vi "MB Serial Master Query Read Input Registers (poly).vi"(0 "VISA resource name":refnum<visa-resource-name>, 1 "Starting Address":u16, 2 "Quantity":u16=1, 4 "Timeout":u32=5000, 5 "error in":errorcluster, 6 "Serial Parameters":T1 {"Slave Address" format="%.0x"}) -> (14 "VISA resource name out":refnum<visa-resource-name>, 15 "Input Registers":u16[](array[numeric]), 16 "Exception Code":u8 format="%.0x", 19 "error out":errorcluster)   [LabVIEW 2011]
doc: "The master uses this VI to read the slaves input registers. This corresponds to a public function code of 4 in the MODBUS protocol."
uses:
  MB Modbus Command.ctl
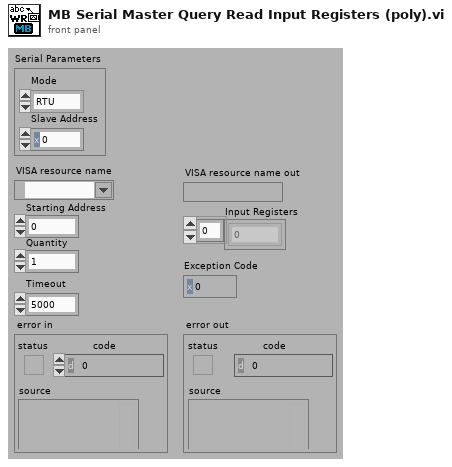
[diagram p1: front panel]
types:
  T1 = cluster{"Mode":enum16{"RTU", "ASCII"}, "Slave Address":u8}
  T2 = typedef "MB Modbus Command.ctl" = cluster{"Function Code":u8, "Starting Address":u16, "Quantity":u16, "Data":u16[], "Discrete":bool[]}
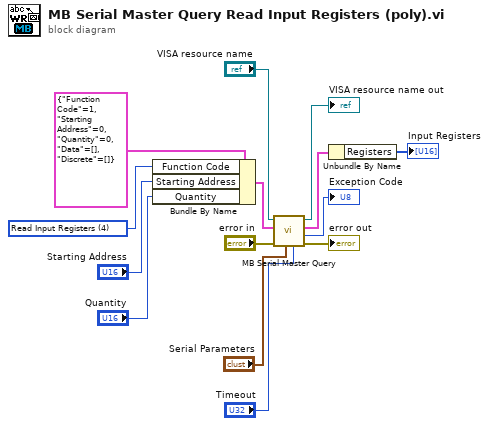
[diagram p0: block diagram]
diagram:
  w11 = u8 4 items=["Read Coils"=1, "Read Discrete Inputs"=2, "Read Holding Registers"=3, "Read Input Registers"=4, "Write Single Coil"=5, "Write Single Register"=6, "Read Exception Status"=7, "Write Multiple Coils"=15, "Write Multiple Registers"=16] ("Function Code")
  n1 = Bundle By Name(cluster=T2 {"Function Code"=1, "Starting Address"=0, "Quantity"=0, "Data"=[], "Discrete"=[]} ("Modbus Command"), "Function Code"=w11, "Starting Address"="Starting Address", "Quantity"="Quantity") -> (w12:T2)
  n2 = call "MB Serial Master Query.vi"("Timeout"="Timeout", "Serial Parameters"="Serial Parameters", "error in (no error)"="error in", "Modbus Command"=w12, "VISA resource name"="VISA resource name") -> ("error out"=→"error out":errorcluster, "Exception Code"=→"Exception Code":u8, "Registers"=w2:cluster{"Registers":u16[], "Discrete":bool[]}, "VISA resource name out"=→"VISA resource name out":refnum<visa-resource-name>)  [unwired: 2 in, 1 out]
  n3 = Unbundle By Name(w2) -> ("Registers"=→"Input Registers":u16[])
